vi "New sequentialLog.vi"(8 "error in":errorcluster, 10 "useDMA (T)":bool=TRUE, 11 "perChannelStreaming (T)":bool=TRUE) -> (0 "error out":errorcluster, 3 "new sequentialLog out":refnum<k24>)   [LabVIEW 2020, in "Ballard_1553_Hardware_ni.lvlib"]
uses:
  Ballard_1553_Hardware_ni.lvlib
  C:/Users/Administrator/Desktop/GIT/Ballard-MIL-STD-1553-Custom-Device/Source/System Explorer/SubVIs/Parse XML Ballard/1.2/BTIXML_SerDes.dll
  Ballard-MIL-STD-1553-Custom-Device/Source/System Explorer/SubVIs/Parse XML Ballard/1.2/BTIXML_SerDes.dll
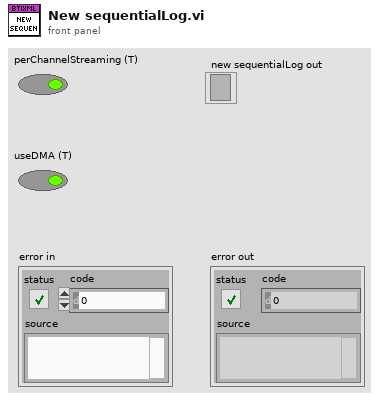
[diagram p1: front panel]
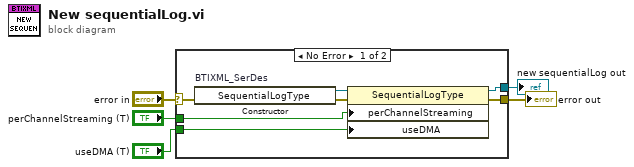
[diagram p0: block diagram]
diagram:
  n1 = case shown="No Error" "error in" {
    selector: "error in" -> [w12 w13]
    tunnel: [w9 w13] -> w4
    tunnel: [w8 _] -> w1
    tunnel: "useDMA (T)" -> [w7 _]
    tunnel: "perChannelStreaming (T)" -> [w6 _]
    frame No Error {
      n2 = constructor on="BTIXML_SerDes" class="SequentialLogType"(error in=w12) -> (reference out=w11:refnum<k24>, error out=w10:errorcluster)  [unwired: 2 in, 1 out]
      n3 = property class="SequentialLogType"(reference=w11, error in=w10, "perChannelStreaming"=w6, "useDMA"=w7) -> (reference out=w8:refnum<k24>, error out=w9:errorcluster)
    }
    frame Error {
    }
  }
  "error out" <- w4
  "new sequentialLog out" <- w1
